vi "read_image.vi"(3 "error in":errorcluster, 4 "header size":i8=10, 5 "connection ID":refnum<k5>) -> (0 "error out":errorcluster, 1 "image data":T1, 2 "connection ID out":refnum<k5>)   [LabVIEW 2018]
uses:
  <vilib>/picture/picture.llb/imagedata.ctl
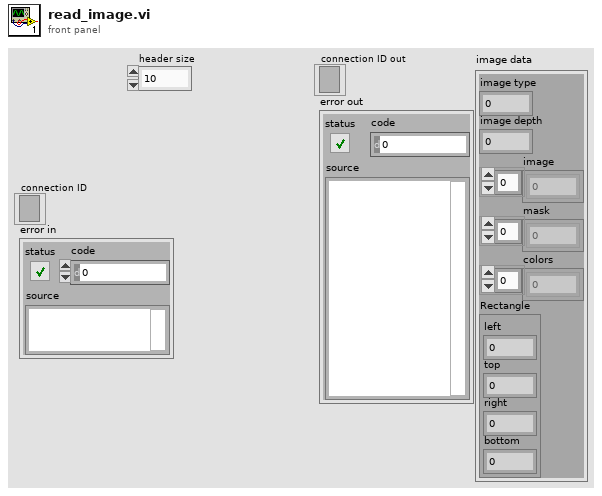
[diagram p1: front panel]
types:
  T1 = typedef "imagedata.ctl" = cluster{"image type":i32, "image depth":i32, "image":u8[], "mask":u8[], "colors":u32[], "Rectangle":cluster{"left":i16, "top":i16, "right":i16, "bottom":i16}}
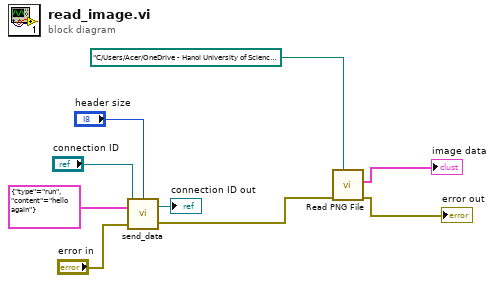
[diagram p0: block diagram]
diagram:
  n1 = call "send_data.vi"("header size"="header size", "error in"="error in", "Cluster"=cluster{"type":string, "content":string} {"type"="run", "content"="hello again"}, "connection ID"="connection ID") -> ("error out"=w3:errorcluster, "connection ID out"=→"connection ID out":refnum<k5>)
  n2 = call <vilib>:"Read PNG File.vi"("error in (no error)"=w3, "path to PNG file"=path "C:/Users/Acer/OneDrive - Hanoi University of Science and Technology/Documents/LabViewProject/Project/labview/image.png") -> ("error out"=→"error out":errorcluster, "image data"=→"image data":T1)  [unwired: 7 in, 1 out]
